vi "Constructor.vi"(8 "error in (no error)":errorcluster, 11 "VISA resource name":refnum<visa-resource-name>) -> (0 "error out":errorcluster, 3 "Line Tracker out":refnum<class "Line Tracker.lvclass">, 5 "User Events":T1)   [LabVIEW 2026, in "Line Tracker.lvlib" / "Line Tracker.lvclass"]
uses:
  Line Tracker.lvclass
  Line Tracker.lvclass/Line Tracker.ctl
  Tracking Values.ctl
  User Events.ctl
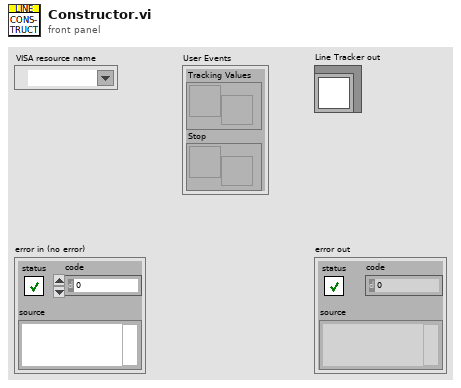
[diagram p1: front panel]
types:
  T1 = typedef "User Events.ctl" = cluster{"Tracking Values":refnum<user-event>, "Stop":refnum<user-event>}
  T2 = typedef "Tracking Values.ctl" = cluster{"LEFT":bool, "CENTRE":bool, "RIGHT":bool}
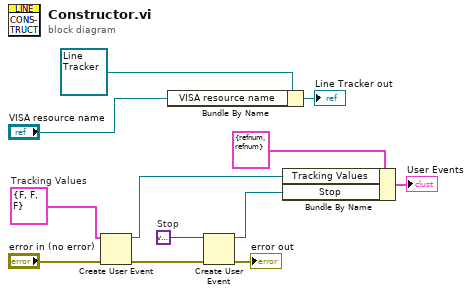
[diagram p0: block diagram]
diagram:
  w8 = variant  # Stop
  w9 = T2 {"LEFT"=FALSE, "CENTRE"=FALSE, "RIGHT"=FALSE}  # Tracking Values
  n1 = Create User Event(user event datatype=w9, error in="error in (no error)") -> (user event=w7:refnum<user-event>, error out=w2:errorcluster)
  n2 = Bundle By Name(cluster=refnum<class "Line Tracker.lvclass"> refnum ("Line Tracker in"), "VISA resource name"="VISA resource name") -> (→"Line Tracker out":refnum<class "Line Tracker.lvclass">)
  n3 = Create User Event(user event datatype=w8, error in=w2) -> (user event=w6:refnum<user-event>, error out=→"error out":errorcluster)
  n4 = Bundle By Name(cluster=T1 {"Tracking Values"=refnum, "Stop"=refnum}, "Tracking Values"=w7, "Stop"=w6) -> (→"User Events":T1)
